vi "WorkorderHandler_TestClassPerformance.vi"() -> ()   [LabVIEW 2011]
doc: "This tests class performance for generating, creating, obtaining, setting and deleting n class objects."
uses:
  Software/DataStructures/WorkorderHandler_ObjectData.ctl
panel:
  in  "error in (no error)":errorcluster
  out "total":u32
  out "Delete Pass":bool
  out "Get Data Modify Pass":bool
  out "Get Data Pass":bool
  in  "Use No Error set data":bool
  out "error out":errorcluster
  in  "Number":i32=1000
  out "delete":u32
  out "set":u32
  out "get":u32
  out "create":u32
  out "generate data":u32
  in  "data":T1
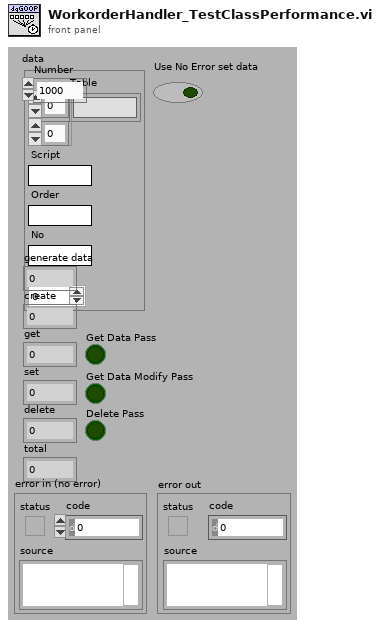
[diagram p1: front panel]
types:
  T1 = typedef "WorkorderHandler_ObjectData.ctl" = cluster{"Table":string[][], "Script":string, "Order":string, "No":string, "Time":dbl}
  T2 = typedef "WorkorderHandler_ObjectReference.ctl" = refnum<k1>
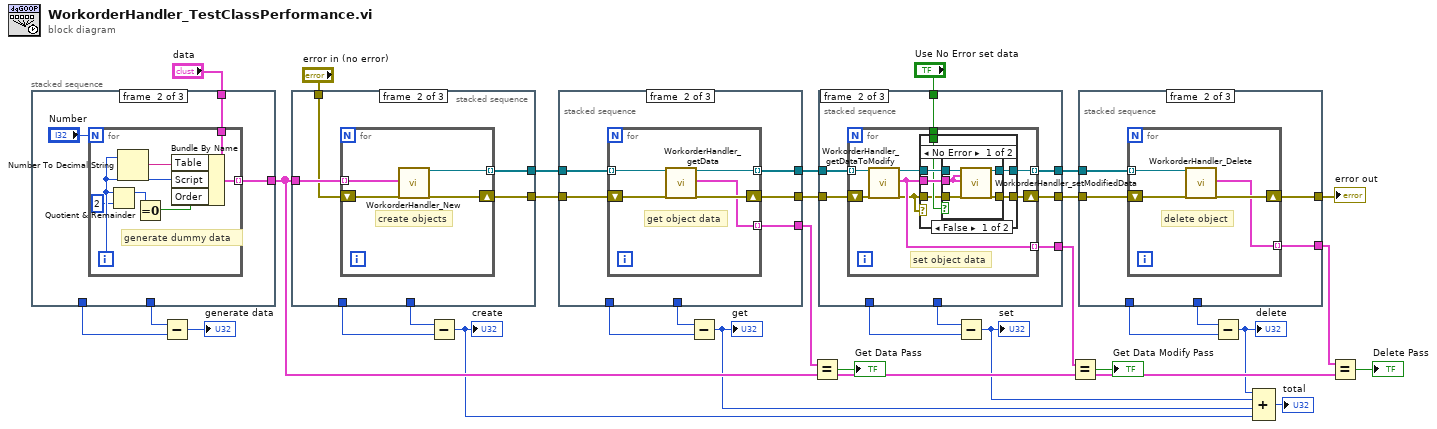
[diagram p0: block diagram]
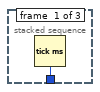
[diagram p2: hidden frame]
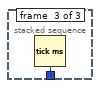
[diagram p3: hidden frame]
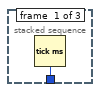
[diagram p4: hidden frame]
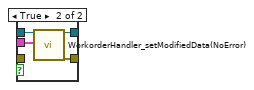
[diagram p5: hidden frame]
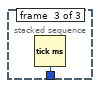
[diagram p7: hidden frame]
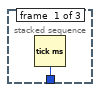
[diagram p8: hidden frame]
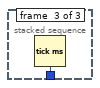
[diagram p9: hidden frame]
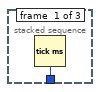
[diagram p10: hidden frame]
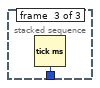
[diagram p11: hidden frame]
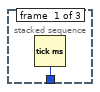
[diagram p12: hidden frame]
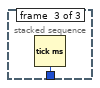
[diagram p13: hidden frame]
diagram:
  n1 = stacked-sequence {
    tunnel: [w34 _ _] -> w30
    tunnel: [_ _ w45] -> w31
    tunnel: [_ w36 _] -> w8
    tunnel: "data" -> [_ w37 _]
    frame #0 {
      n2 = Tick Count (ms)() -> (millisecond timer value=w34:u32)
    }
    frame #1 {
      n3 = for {
        N: "Number" -> [_]
        tunnel: w37 -> [w44]
        tunnel: [w43] -> w36 mode=indexing
        i -> [w41]
        # "generate dummy data"
        n4 = Quotient & Remainder(x=w41, y=2) -> (x-y*floor(x/y)=w39:i32)  [unwired: 1 out]
        n5 = Number To Decimal String(number=w41) -> (decimal integer string=w42:string)  [unwired: 1 out]
        n6 = Equal To 0?(x=w39) -> (x = 0?=w38:bool)
        n7 = Bundle By Name(cluster=w44, "Table"=w42, "Script"=w41, "Order"=w38) -> (w43:T1)
      }
    }
    frame #2 {
      n8 = Tick Count (ms)() -> (millisecond timer value=w45:u32)
    }
  }
  n9 = Subtract(x=w31, y=w30) -> (x-y=→"generate data":u32)
  n10 = stacked-sequence {
    tunnel: [w46 _ _] -> w33
    tunnel: [_ _ w55] -> w32
    tunnel: w8 -> [_ w50 _]
    tunnel: [_ w49 _] -> w23
    tunnel: [_ w48 _] -> w20
    tunnel: "error in (no error)" -> [_ w47 _]
    frame #0 {
      n11 = Tick Count (ms)() -> (millisecond timer value=w46:u32)
    }
    frame #1 {
      n12 = for {
        shift-right: [w53] -> w49
        shift-left: w47 -> [w54]
        tunnel: w50 -> [w52] mode=indexing
        tunnel: [w51] -> w48 mode=indexing
        # "create objects"
        n13 = call "WorkorderHandler_New.vi"("data"=w52, "error in (no error)"=w54) -> ("reference"=w51:T2, "error out"=w53:errorcluster)  [unwired: 16 out]
      }
    }
    frame #2 {
      n14 = Tick Count (ms)() -> (millisecond timer value=w55:u32)
    }
  }
  n15 = Subtract(x=w32, y=w33) -> (x-y=w3:u32)
  "create" <- w3
  n16 = stacked-sequence {
    tunnel: [w56 _ _] -> w29
    tunnel: [_ _ w67] -> w28
    tunnel: w23 -> [_ w61 _]
    tunnel: [_ w60 _] -> w22
    tunnel: w20 -> [_ w59 _]
    tunnel: [_ w58 _] -> w19
    tunnel: [_ w57 _] -> w13
    frame #0 {
      n17 = Tick Count (ms)() -> (millisecond timer value=w56:u32)
    }
    frame #1 {
      n18 = for {
        shift-right: [w65] -> w60
        shift-left: w61 -> [w66]
        tunnel: w59 -> [w64] mode=indexing
        tunnel: [w63] -> w58 mode=indexing
        tunnel: [w62] -> w57 mode=indexing
        # "get object data"
        n19 = call "WorkorderHandler_getData.vi"("reference"=w64, "error in (no error)"=w66) -> ("duplicate reference"=w63:T2, "data"=w62:T1, "error out"=w65:errorcluster)  [unwired: 1 in, 14 out]
      }
    }
    frame #2 {
      n20 = Tick Count (ms)() -> (millisecond timer value=w67:u32)
    }
  }
  n21 = Subtract(x=w28, y=w29) -> (x-y=w4:u32)
  "get" <- w4
  n22 = Equal?(x=w13, y=w8) -> (x = y?=→"Get Data Pass":bool)
  n23 = stacked-sequence {
    tunnel: [w68 _ _] -> w27
    tunnel: [_ _ w100] -> w26
    tunnel: w22 -> [_ w74 _]
    tunnel: [_ w73 _] -> w21
    tunnel: w19 -> [_ w72 _]
    tunnel: [_ w71 _] -> w18
    tunnel: "Use No Error set data" -> [_ w70 _]
    tunnel: [_ w69 _] -> w9
    frame #0 {
      n24 = Tick Count (ms)() -> (millisecond timer value=w68:u32)
    }
    frame #1 {
      n25 = for {
        shift-right: [w82] -> w73
        shift-left: w74 -> [w78]
        tunnel: w72 -> [w80] mode=indexing
        tunnel: [w81] -> w71 mode=indexing
        tunnel: w70 -> [w77]
        tunnel: [w76] -> w69 mode=indexing
        # "set object data"
        n26 = call "WorkorderHandler_getDataToModify.vi"("reference"=w80, "error in (no error)"=w78) -> ("duplicate reference"=w79:T2, "data"=w76:T1, "error out"=w75:errorcluster)  [unwired: 1 in, 14 out]
        n27 = case shown="No Error" w75 {
          tunnel: [w88 w98] -> w82
          tunnel: [w87 w99] -> w81
          tunnel: w79 -> [w86 w99]
          tunnel: w76 -> [w85 _]
          tunnel: w77 -> [w84 _]
          tunnel: w75 -> [w83 w98]
          frame No Error {
            n28 = case shown="False" w84 {
              tunnel: w83 -> [w93 _]
              tunnel: [w92 w95] -> w88
              tunnel: [w91 w97] -> w87
              tunnel: w86 -> [w90 w96]
              tunnel: w85 -> [w89 w94]
              frame False {
                n29 = call "WorkorderHandler_setModifiedData.vi"("reference"=w90, "data (unmodified)"=w89, "data"=w89, "error in (no error)"=w93) -> ("duplicate reference"=w91:T2, "error out"=w92:errorcluster)  [unwired: 14 out]
              }
              frame True {
                n30 = call "WorkorderHandler_setModifiedData(NoError).vi"("reference"=w96, "data"=w94) -> ("duplicate reference"=w97:T2, "error out"=w95:errorcluster)  [unwired: 16 out]
              }
            }
          }
          frame Error {
          }
        }
      }
    }
    frame #2 {
      n31 = Tick Count (ms)() -> (millisecond timer value=w100:u32)
    }
  }
  n32 = Subtract(x=w26, y=w27) -> (x-y=w5:u32)
  "set" <- w5
  n33 = Equal?(x=w9, y=w8) -> (x = y?=→"Get Data Modify Pass":bool)
  n34 = stacked-sequence {
    tunnel: [w101 _ _] -> w25
    tunnel: [_ _ w110] -> w24
    tunnel: w21 -> [_ w105 _]
    tunnel: w18 -> [_ w104 _]
    tunnel: [_ w103 _] -> w15
    tunnel: [_ w102 _] -> w7
    frame #0 {
      n35 = Tick Count (ms)() -> (millisecond timer value=w101:u32)
    }
    frame #1 {
      n36 = for {
        shift-right: [w108] -> w103
        shift-left: w105 -> [w109]
        tunnel: w104 -> [w107] mode=indexing
        tunnel: [w106] -> w102 mode=indexing
        # "delete object"
        n37 = call "WorkorderHandler_Delete.vi"("reference"=w107, "error in (no error)"=w109) -> ("data"=w106:T1, "error out"=w108:errorcluster)  [unwired: 1 in, 15 out]
      }
    }
    frame #2 {
      n38 = Tick Count (ms)() -> (millisecond timer value=w110:u32)
    }
  }
  "error out" <- w15
  n39 = Subtract(x=w24, y=w25) -> (x-y=w6:u32)
  "delete" <- w6
  n40 = Compound Arithmetic op=ADD(w6, w5, w4, w3) -> (→"total":u32)
  n41 = Equal?(x=w7, y=w8) -> (x = y?=→"Delete Pass":bool)
